vi "Typecast.vi"() -> ()   [LabVIEW 2011]
panel:
  out "output 1":enum16{"do", "test"}(ring)
  in  "Enum":enum16{"do", "test"}(ring)
  out "index":i32
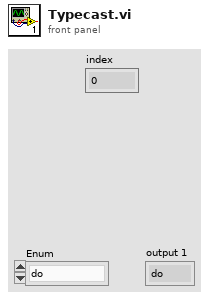
[diagram p1: front panel]
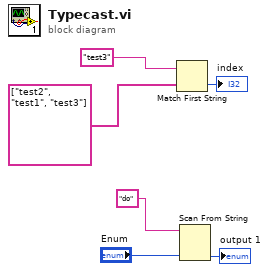
[diagram p0: block diagram]
diagram:
  n1 = Match First String(2:string[] ["test2", "test1", "test3"] ("string array"), 3:"test3" ("string")) -> (0:→"index":i32)  [unwired: 1 out]
  n2 = Scan From String(input string="do" ("format string"), default 1="Enum") -> (output 1=→"output 1":enum16{"do", "test"})  [unwired: 3 in, 3 out]
